vi "test1-LocalExternalStatusRegistration.vi"(8 "error in (no error)":errorcluster, 11 "TestCase in":refnum<class "testcase-CSMBroadcast.lvclass">) -> (0 "error out":errorcluster, 3 "TestCase out":refnum<class "testcase-CSMBroadcast.lvclass">)   [LabVIEW 2017, in "testcase-CSMBroadcast.lvclass"]
uses:
  testcase-CSMBroadcast.lvclass
  0b17d103-e67b-41be-a9eb-a2ee1311ff1f.vi
  5999693e-4f8a-4b34-ae87-f34dff5771be.vi
  52a2a10a-a04b-4bad-8df4-e1eb944f47cc.vi
  826f03dd-b4b5-4c6b-9085-8edf6da4f43b.vi
  src/user.lib/_NEVSTOP/Communicable State Machine(CSM)/AdvanceAPI/CSM - Revert Arguments-Safe String.vi
  src/user.lib/_NEVSTOP/Communicable State Machine(CSM)/AdvanceAPI/CSM - Make String Arguments Safe.vi
  src/user.lib/_NEVSTOP/Communicable State Machine(CSM)/AdvanceAPI/CSM - Break Down Multiple States String.vi
  src/user.lib/_NEVSTOP/Communicable State Machine(CSM)/AdvanceAPI/CSM - Keywords.vi
  src/user.lib/_NEVSTOP/Communicable State Machine(CSM)/_Polymophic/CSM - Replace Marks in Messages.vi
  src/user.lib/_NEVSTOP/Communicable State Machine(CSM)/AdvanceAPI/CSM - Get Module Attribute.vi
  src/user.lib/_NEVSTOP/Communicable State Machine(CSM)/_Shared/Trim Single-line Text.vi
  <vilib>/addons/_JKI Toolkits/VI Tester/TestCase.llb/TestCase.lvclass
  src/user.lib/_NEVSTOP/Communicable State Machine(CSM)/Communicable State Machine.lvlib
  C:/Program Files (x86)/National Instruments/LabVIEW 2017/vi.lib/addons/_JKI Toolkits/VI Tester/TestCase.llb/TestCase.lvclass
panel:
  out "One-Shot Unregistrations":string
  out "Waited (ms)":u32
  out "One-Shot Registrations":string
  out "LoopCount 2":i32
  out "State History":string
  out "LoopCount":i32
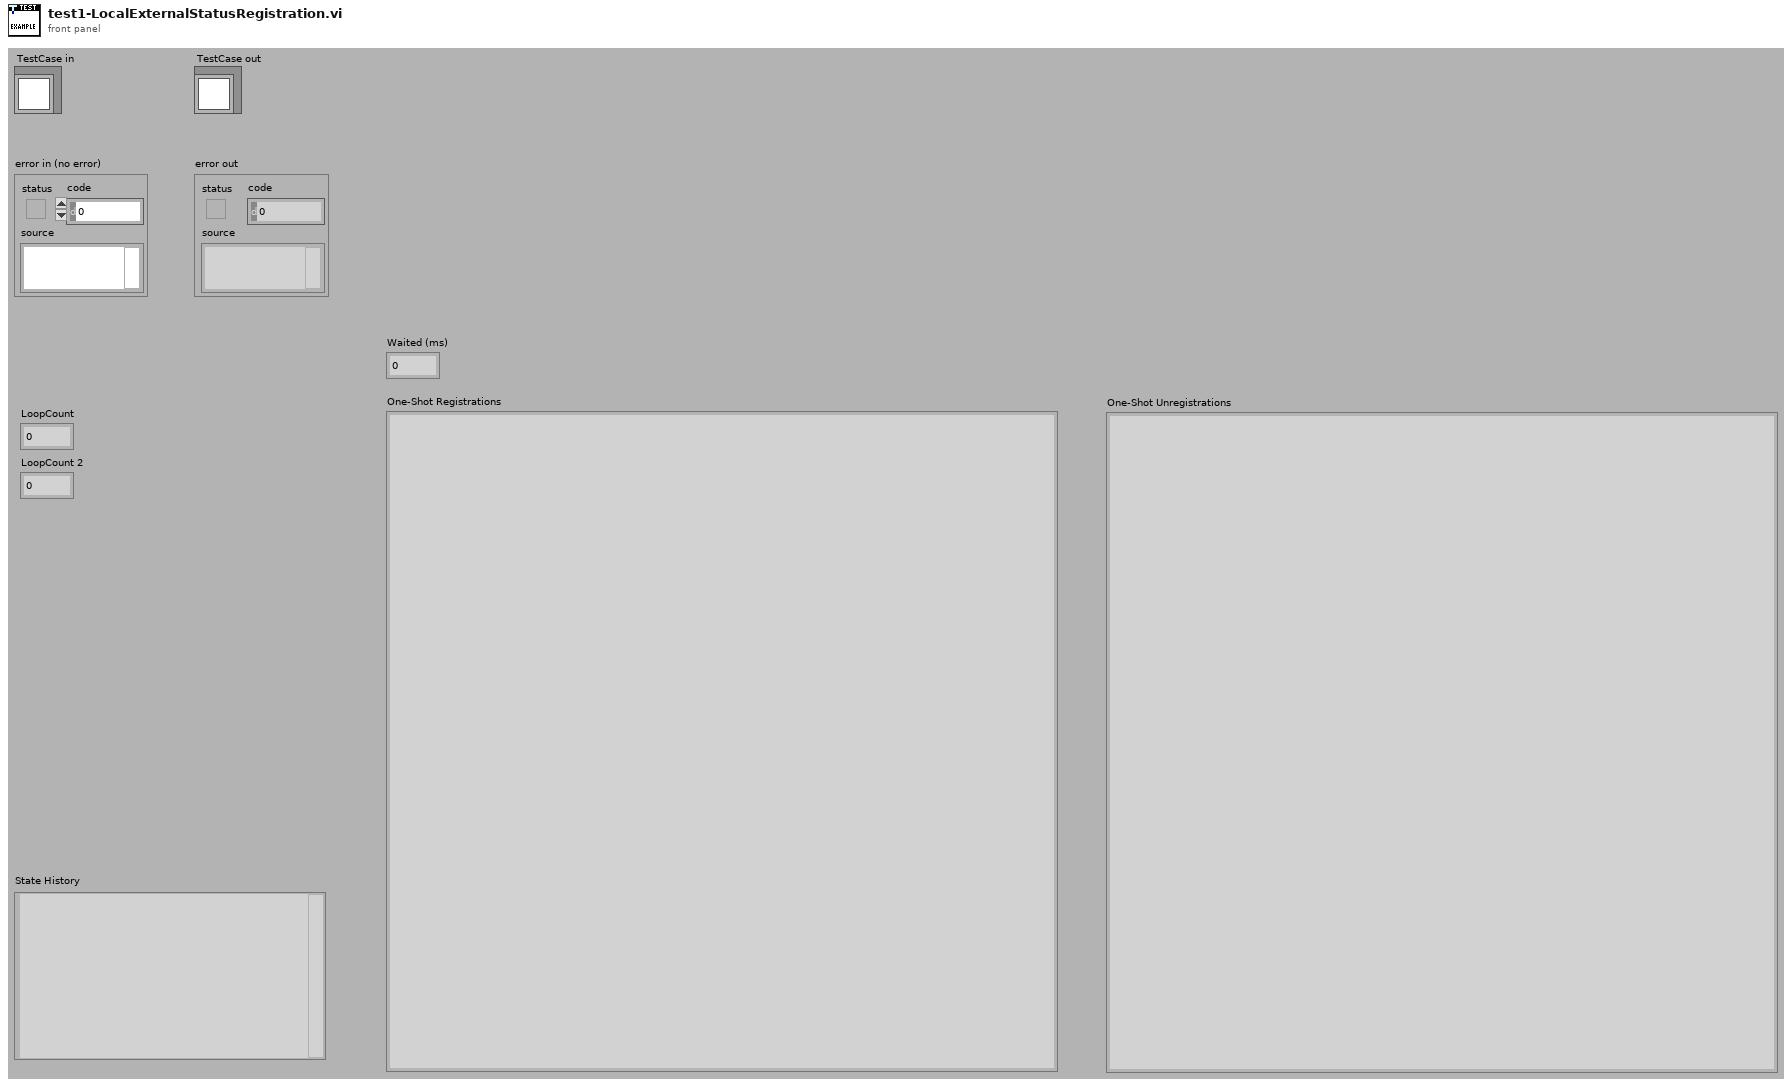
[diagram p1: front panel]
types:
  T1 = enum32{"Invalid", "Standard", "Closed", "Hidden", "Minimized", "Maximized"}
  T2 = enum32{"invalid app kind", "Development System", "Run Time System", "Student Edition", "Embedded LabVIEW", "Evaluation", "Custom"}
  T3 = typedef "Communicable State Machine.lvlib/_CSM_Response Source Message.ctl" = cluster{"‘State":string, "’Arguments":string, "’Error":errorcluster}
  T4 = cluster{"Current VI Reference":refnum<vi>, "Close Panel on Exit?":bool}
  T5 = cluster{"Core":cluster{"Current VI Reference":refnum<vi>, "Close Panel on Exit?":bool}, "Your Boolean data":bool, "Your string data":string}
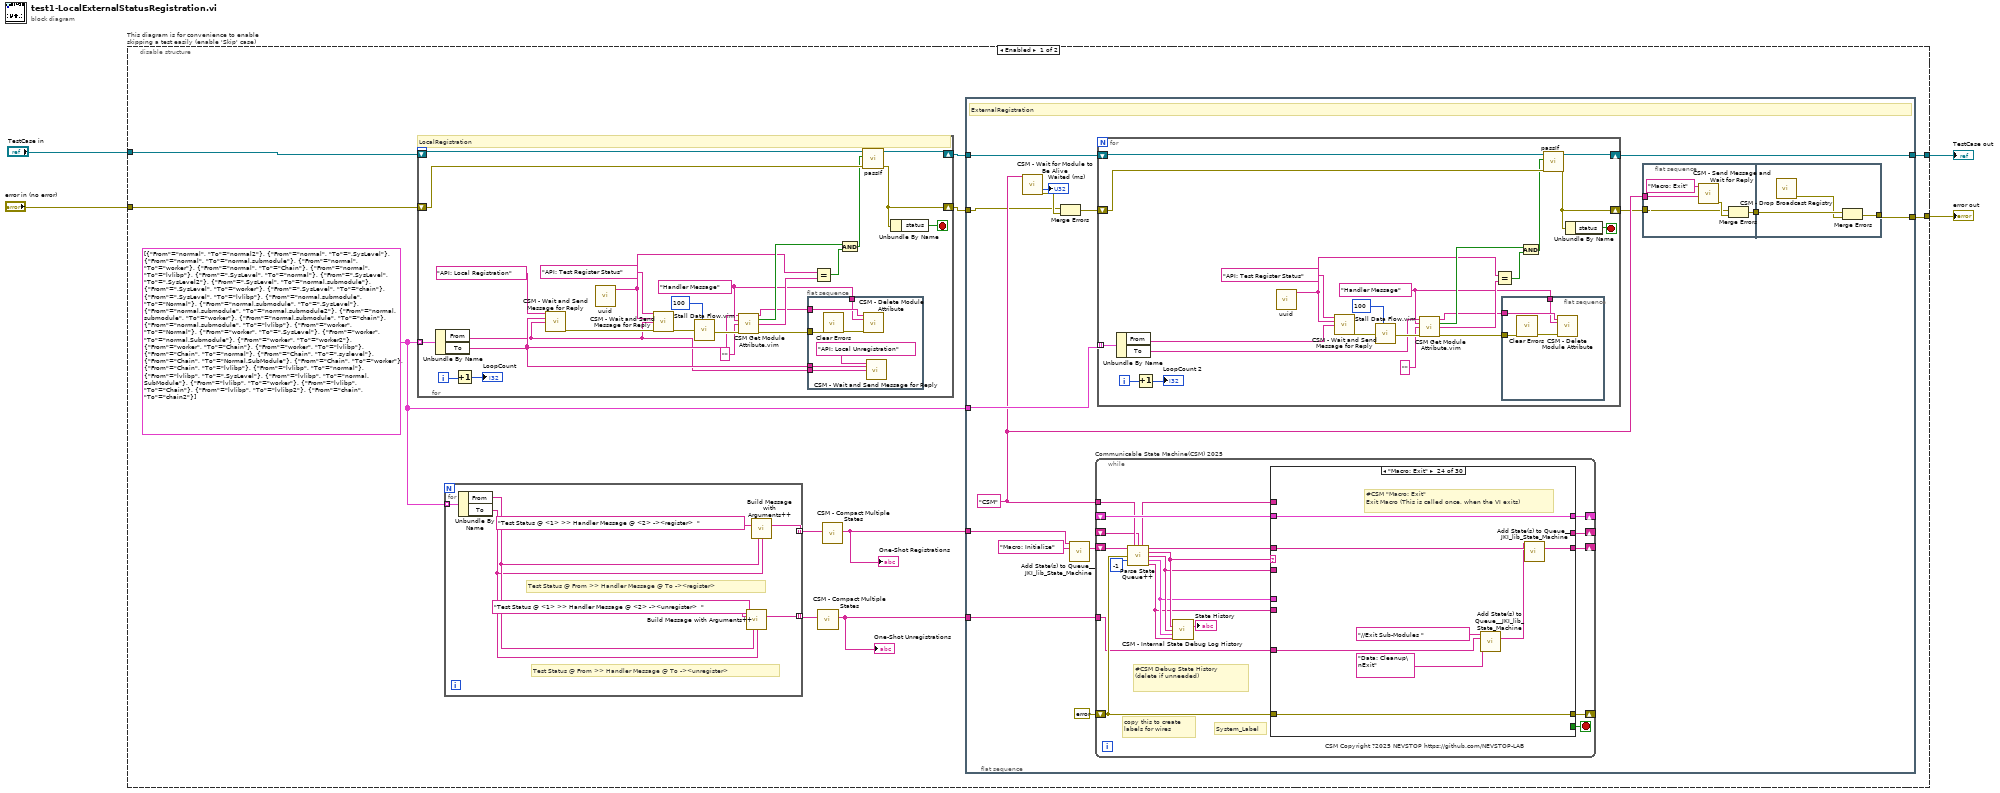
[diagram p0: block diagram]
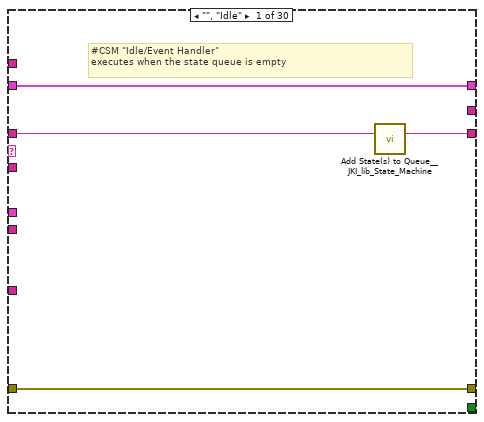
[diagram p2: hidden frame]
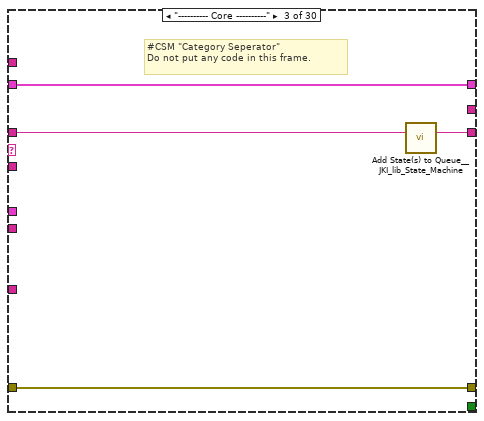
[diagram p4: hidden frame]
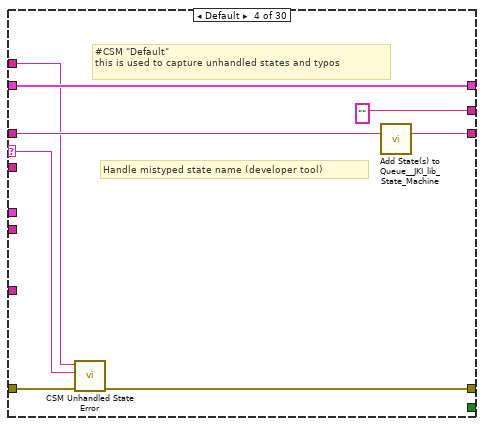
[diagram p5: hidden frame]
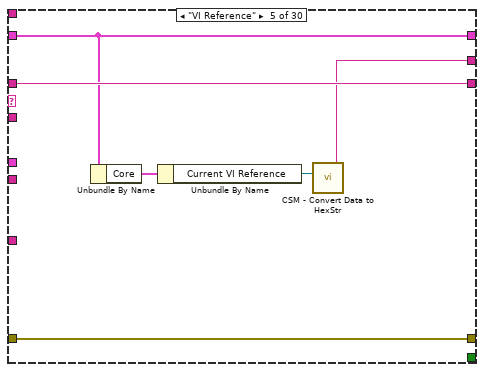
[diagram p6: hidden frame]
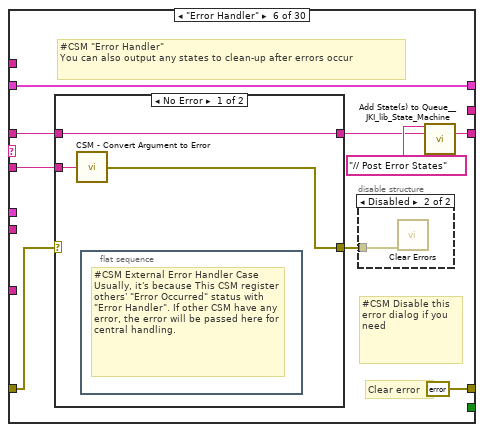
[diagram p7: hidden frame]
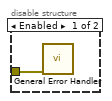
[diagram p8: hidden frame]
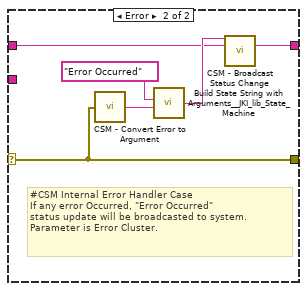
[diagram p9: hidden frame]
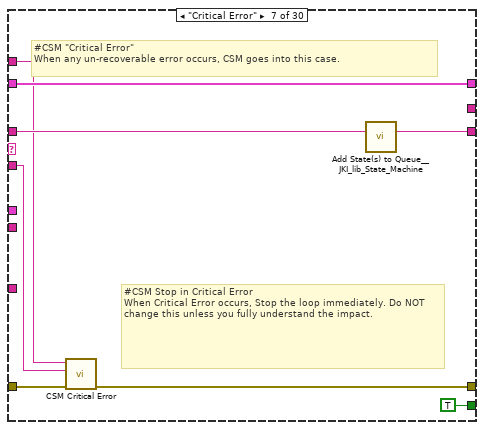
[diagram p10: hidden frame]
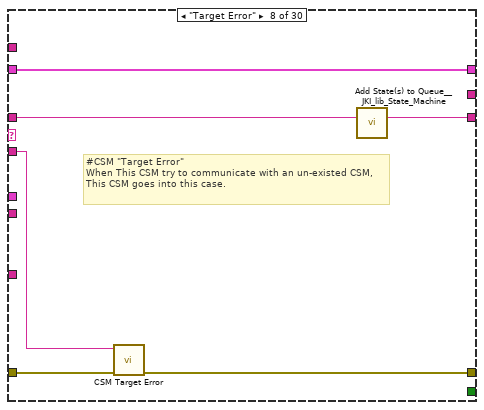
[diagram p11: hidden frame]
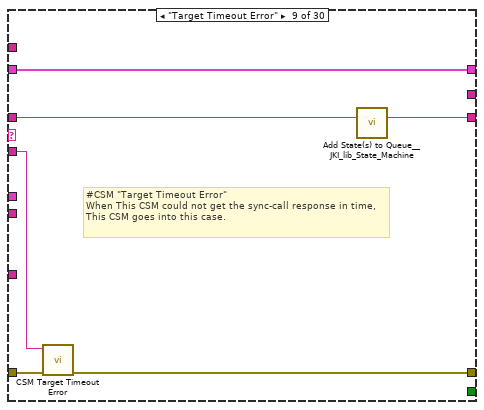
[diagram p12: hidden frame]
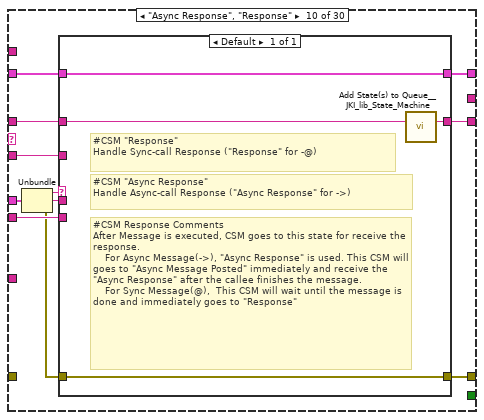
[diagram p13: hidden frame]
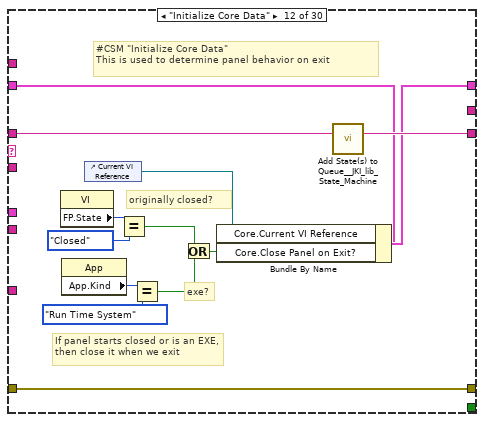
[diagram p15: hidden frame]
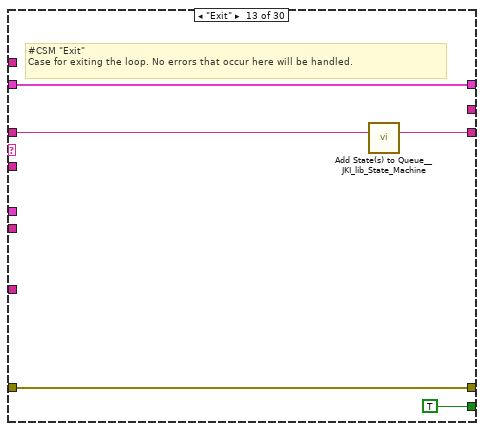
[diagram p16: hidden frame]
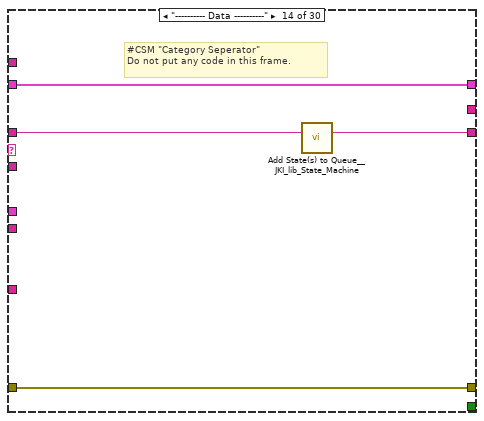
[diagram p17: hidden frame]
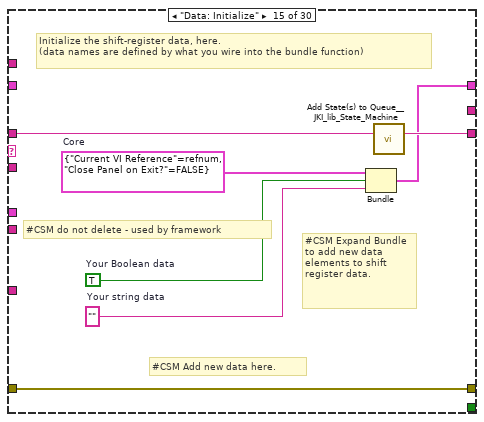
[diagram p18: hidden frame]
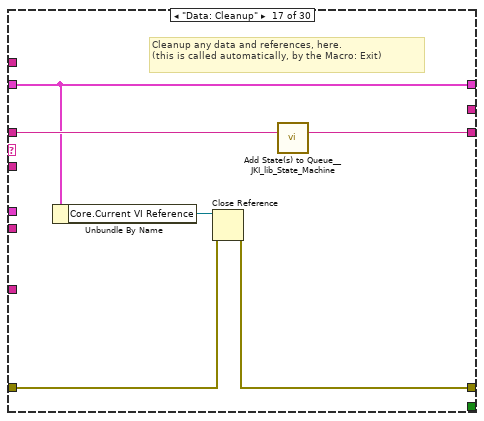
[diagram p20: hidden frame]
diagram:
  n1 = disable-structure "This diagram is for convenience to enable skipping a test easily (enable 'Skip' case)" shown="Enabled" {
    disable-tunnel: "TestCase in" -> [w14 w386]
    disable-tunnel: [w12 w384] -> w1
    disable-tunnel: [w5 w385] -> w3
    disable-tunnel: "error in (no error)" -> [w15 w383]
    frame Enabled {
      w10 = cluster{"From":string, "To":string}[] [{"From"="normal", "To"="normal2"}, {"From"="normal", "To"=".SysLevel"}, {"From"="normal", "To"="normal.submodule"}, {"From"="normal", "To"="worker"}, {"From"="normal", "To"="Chain"}, {"From"="normal", "To"="lvlibp"}, {"From"=".SysLevel", "To"="normal"}, {"From"=".SysLevel", "To"=".SysLevel2"}, {"From"=".SysLevel", "To"="normal.submodule"}, {"From"=".SysLevel", "To"="worker"}, {"From"=".SysLevel", "To"="chain"}, {"From"=".SysLevel", "To"="lvlibp"}, {"From"="normal.submodule", "To"="Normal"}, {"From"="normal.submodule", "To"=".SysLevel"}, {"From"="normal.submodule", "To"="normal.submodule2"}, {"From"="normal.submodule", "To"="worker"}, {"From"="normal.submodule", "To"="chain"}, {"From"="normal.submodule", "To"="lvlibp"}, {"From"="worker", "To"="Normal"}, {"From"="worker", "To"=".SysLevel"}, {"From"="worker", "To"="normal.Submodule"}, {"From"="worker", "To"="worker2"}, {"From"="worker", "To"="Chain"}, {"From"="worker", "To"="lvlibp"}, {"From"="Chain", "To"="normal"}, {"From"="Chain", "To"=".syslevel"}, {"From"="Chain", "To"="Normal.SubModule"}, {"From"="Chain", "To"="worker"}, {"From"="Chain", "To"="lvlibp"}, {"From"="lvlibp", "To"="normal"}, {"From"="lvlibp", "To"=".SysLevel"}, {"From"="lvlibp", "To"="normal.SubModule"}, {"From"="lvlibp", "To"="worker"}, {"From"="lvlibp", "To"="Chain"}, {"From"="lvlibp", "To"="lvlibp2"}, {"From"="chain", "To"="chain2"}]
      n2 = for {
        shift-right: [w24] -> w11
        shift-left: w15 -> [w25]
        shift-right: [w26] -> w13
        shift-left: w14 -> [w27]
        tunnel: w10 -> [w38] mode=indexing
        i -> [w40]
        stop <- w23 stop-if-true
        w18 = "Handler Message" ("To")
        # "LocalRegistration"
        n3 = Unbundle By Name(w38) -> ("From"=w16:string, "To"=w17:string)
        n4 = Increment(x=w40) -> (x+1=→"LoopCount":i32)
        n5 = call "CSM - Wait and Send Message for Reply.vi"("State"="API: Local Registration", "Arguments (\"\")"=w17, "Target Module"=w16) -> ("error out"=w35:errorcluster)  [unwired: 9 in, 3 out]
        n6 = call "uuid.vi"() -> ("UUID"=w29:string)  [unwired: 11 in]
        n7 = call "CSM - Wait and Send Message for Reply.vi"("State"="API: Test Register Status", "Arguments (\"\")"=w29, "Target Module"=w16, "Error In (No Error)"=w35) -> ("error out"=w34:errorcluster)  [unwired: 8 in, 3 out]
        n8 = call "Stall Data Flow.vim"("value in"=w34, "milliseconds to wait"=u32 100) -> ("value out"=w32:errorcluster)  [unwired: 1 out]
        n9 = call "CSM Get Module Attribute.vim"("CSM Name"=w17, "Attribute"=w18, "Default Value (Empty Variant)"="", "Error In"=w32) -> ("CSM Name (Dup)"=w19:string, "Found"=w31:bool, "Value"=w28:string, "error out"=w20:errorcluster)  [unwired: 7 in, 1 out]
        n10 = flat-sequence {
          tunnel: w20 -> [w46]
          tunnel: w19 -> [w45]
          tunnel: w18 -> [w44]
          tunnel: w17 -> [w42]
          tunnel: w16 -> [w41]
          frame #0 {
            n11 = call <vilib>:"Clear Errors.vi"("error in (no error)"=w46) -> ("error out"=w47:errorcluster)  [unwired: 5 in, 1 out]
            n12 = call "CSM - Delete Module Attribute.vi"("CSM Name"=w45, "Attribute"=w44, "Error In"=w47) -> ()  [unwired: 9 in, 4 out]
            n13 = call "CSM - Wait and Send Message for Reply.vi"("State"="API: Local Unregistration", "Arguments (\"\")"=w42, "Target Module"=w41) -> ()  [unwired: 9 in, 4 out]
          }
        }
        n14 = Equal?(x=w29, y=w28) -> (x = y?=w22:bool)
        n15 = And(x=w31, y=w22) -> (x .and. y?=w21:bool)
        n16 = call-dynamic "passIf.vi"("error in (no error)"=w25, "pass"=w21, "TestCase in"=w27) -> ("error out"=w24:errorcluster, "TestCase out"=w26:refnum<class "testcase-CSMBroadcast.lvclass">)  [unwired: 7 in]
        n17 = Unbundle By Name(w24) -> ("status"=w23:bool)
      }
      n18 = for {
        tunnel: w10 -> [w53] mode=indexing
        tunnel: [w52] -> w9 mode=indexing
        tunnel: [w48] -> w7 mode=indexing
        # "Test Status @ From >> Handler Message @ To -><unregister>"
        # "Test Status @ From >> Handler Message @ To -><register>"
        n19 = Unbundle By Name(w53) -> ("From"=w50:string, "To"=w49:string)
        n20 = call-poly "Build Message with Arguments++.vi"("States With Replace Token"="Test Status @ <1> >> Handler Message @ <2> -><unregister>  " ("State"), "<1>"=w50, "<2>"=w49) -> ("States"=w48:string)  [unwired: 12 in]
        n21 = call-poly "Build Message with Arguments++.vi"("States With Replace Token"="Test Status @ <1> >> Handler Message @ <2> -><register>  " ("State"), "<1>"=w50, "<2>"=w49) -> ("States"=w52:string)  [unwired: 12 in]
      }
      n22 = call "CSM - Compact Multiple States.vi"("Multiple States"=w7) -> ("States"=w6:string)  [unwired: 9 in]
      "One-Shot Unregistrations" <- w6
      n23 = call "CSM - Compact Multiple States.vi"("Multiple States"=w9) -> ("States"=w8:string)  [unwired: 9 in]
      "One-Shot Registrations" <- w8
      n24 = flat-sequence {
        tunnel: w13 -> [w67]
        tunnel: [w66] -> w12
        tunnel: w11 -> [w59]
        tunnel: w10 -> [w65]
        tunnel: w8 -> [w63]
        tunnel: w6 -> [w57]
        tunnel: [w55] -> w5
        frame #0 {
          w62 = "CSM" ("Name (\"\" to Use UUID)")
          # "ExternalRegistration"
          n25 = call "CSM - Wait for Module to Be Alive.vi"("CSM Name"=w62) -> ("Waited (ms)"=→"Waited (ms)":u32, "error out"=w64:errorcluster)  [unwired: 12 in, 1 out]
          n26 = Merge Errors(w59, w64) -> (w60:errorcluster)
          n27 = call <vilib>:"Add State(s) to Queue__JKI_lib_State_Machine.vi"("State(s) in Front (\"\")"=w63, "State(s) in (\"\")"="Macro: Initialize" ("Init State(\"Macro: Initialize\")")) -> ("States Out"=w68:string)  [unwired: 13 in]
          n28 = while "Communicable State Machine(CSM) 2025" {
            shift-right: [w119] -> _
            shift-left: _ -> [w118]
            shift-right: [w122] -> _
            shift-left: errorcluster {"status"=FALSE, "code"=0, "source"=""} ("error out") -> [w117]
            shift-right: [w121] -> _
            shift-left: w68 -> [w123]
            tunnel: w62 -> [w115]
            shift-right: [w116] -> _
            shift-left: _ -> [w109]
            tunnel: w57 -> [w106]
            stop <- w120 stop-if-true
            # "#CSM Debug State History\n(delete if unneeded)"
            # "copy this to create labels for wires"
            # "System_Label"
            # "CSM Copyright ?2025 NEVSTOP https://github.com/NEVSTOP-LAB"
            n29 = call "Parse State Queue++.vi"("State Queue"=w123, "Name (\"\" to Use UUID)"=w115, "Response Arguments"=w109, "Previous Error"=w117, "Dequeue (1 ms)"=-1 ("Timeout")) -> ("Name Used"=w110:string, "Remaining States"=w124:string, "Current State"=w114:string, "Arguments"=w113:string, "Additional Information"=w112:T3, "Source CSM"=w111:string)  [unwired: 5 in]
            n30 = call "CSM - Internal State Debug Log History.vi"("State"=w114, "Arguments (\"\")"=w113, ">> Response Source Message >>"=w112, "Source (\"\")"=w111) -> ("Debug Log"=→"State History":string)  [unwired: 11 in]
            n31 = case shown="\"Macro: Exit\"" w114 {
              selector: w114 -> [_ _ _ w138 _ _ _ _ _ _ _ _ _ _ _ _ _ _ _ _ _ _ _ _ _ _ _ _ _ _]
              tunnel: w124 -> [w125 w130 w135 w142 w148 w154 w175 w181 w187 w195 w206 w220 w225 w229 w236 w238 w245 w249 w253 w259 w274 w343 w348 w356 w358 w362 w367 w374 w378 w382]
              tunnel: w113 -> [_ _ _ _ _ w153 w171 w180 w185 w194 _ _ _ _ _ _ _ _ _ w254 w268 _ _ _ _ _ w365 _ _ _]
              tunnel: w118 -> [w126 w129 w132 w140 w147 w157 w176 w182 w188 w197 w205 w213 w223 w226 _ w237 w240 w246 w251 w257 w270 w340 w345 w353 w357 w361 w366 w371 w375 w379]
              tunnel: [w127 w131 w133 w136 w149 errorcluster {"status"=FALSE, "code"=0, "source"=""} ("error out") w172 w178 w184 w200 w207 w217 w222 w227 w233 w239 w241 w247 w250 w255 w271 w341 w346 w354 w359 w363 w368 w372 w376 w380] -> w122
              tunnel: w117 -> [w127 w131 w133 w143 w149 w155 w177 w179 w186 _ w207 w217 w222 w227 w233 w239 w242 w247 w250 w256 w272 w341 w346 w354 w359 w363 w368 w372 w376 w380]
              tunnel: [w128 w130 w134 w141 w148 w150 w174 w183 w189 w196 w206 w219 w224 w228 w235 w238 w244 w248 w252 w258 w273 w342 w347 w355 w358 w362 w367 w373 w377 w381] -> w121
              tunnel: [_ _ _ _ _ _ TRUE _ _ _ _ _ TRUE _ _ _ _ _ _ _ _ _ _ _ _ _ _ _ _ _] -> w120
              tunnel: [w126 w129 w132 w140 w147 w157 w176 w182 w188 w198 w205 w218 w223 w226 w234 w237 w240 w246 w251 w257 w270 w340 w345 w353 w357 w361 w366 w371 w375 w379] -> w119
              tunnel: w111 -> [_ _ _ _ _ _ _ _ _ w192 _ _ _ _ _ _ _ _ _ _ _ _ _ _ _ _ _ _ _ _]
              tunnel: w112 -> [_ _ _ _ _ _ _ _ _ w199 _ _ _ _ _ _ _ _ _ _ _ _ _ _ _ _ _ _ _ _]
              tunnel: [_ _ _ "" w144 _ _ _ _ _ _ _ _ _ _ _ _ _ _ _ _ _ _ _ _ "API1 Response" w364 _ _ _] -> w116
              tunnel: w110 -> [_ _ _ w137 _ _ w170 _ _ _ _ _ _ _ _ _ _ _ _ _ _ _ _ _ _ _ _ _ _ _]
              tunnel: w106 -> [_ _ _ _ _ _ _ _ _ _ _ _ _ _ _ _ _ _ _ _ _ _ _ w349 _ _ _ _ _ _]
              frame "", "Idle" {
                # "#CSM \"Idle/Event Handler\"\nexecutes when the state queue is empty"
                n32 = call <vilib>:"Add State(s) to Queue__JKI_lib_State_Machine.vi"("State(s) in (\"\")"=w125) -> ("States Out"=w128:string)  [unwired: 14 in]
              }
              frame "CSM Documentation" {
                # "#CSM README FIRST\n\nCommunicable State Machine(CSM) is a LabVIEW application framework that builds upon JKI State Machine(JKISM). It follows the pattern of JKISM and extends the keywords to describe message communication between modules, including concepts such as Sync-Message, Async-Message, Subscription/Unsubscription of status - essential elements for creating reusable code modules. For more information, please visit the CSM wiki: https://nevstop-lab.github.io/CSM-Wiki/\n\nFor instructions on JKI State Machine, visit: http://jki.net/state-machine/\nFor information about CSM, visit: https://github.com/NEVSTOP-LAB"
                # "#CSM \"Documentation\"\nCase for holding CSM Documenation"
              }
              frame "---------- Core ----------" {
                # "#CSM \"Category Seperator\"\nDo not put any code in this frame."
                n33 = call <vilib>:"Add State(s) to Queue__JKI_lib_State_Machine.vi"("State(s) in (\"\")"=w135) -> ("States Out"=w134:string)  [unwired: 14 in]
              }
              frame Default {
                # "#CSM \"Default\"\nthis is used to capture unhandled states and typos"
                # "Handle mistyped state name (developer tool)"
                n34 = call "CSM Unhandled State Error.vi"("error in (no error)"=w143, "Undefined State"=w138, "CSM Name"=w137) -> ("error out"=w136:errorcluster)  [unwired: 8 in]
                n35 = call <vilib>:"Add State(s) to Queue__JKI_lib_State_Machine.vi"("State(s) in (\"\")"=w142) -> ("States Out"=w141:string)  [unwired: 14 in]
              }
              frame "VI Reference" {
                n36 = Unbundle By Name(w147) -> ("Core"=w146:T4)
                n37 = Unbundle By Name(w146) -> ("Current VI Reference"=w145:refnum<vi>)
                n38 = call "CSM - Convert Data to HexStr.vi"("Variant"=w145) -> ("HEX String (0-9,A-F)"=w144:string)  [unwired: 8 in]
              }
              frame "Error Handler" {
                # "#CSM Disable this error dialog if you need"
                # "#CSM \"Error Handler\"\nYou can also output any states to clean-up after errors occur"
                # "Clear error"
                n39 = case shown="No Error" w155 {
                  selector: w155 -> [_ w164]
                  tunnel: [w163 w166] -> w151
                  tunnel: w154 -> [w163 w165]
                  tunnel: w153 -> [w162 _]
                  tunnel: [w161 w164] -> w156
                  frame No Error {
                    n40 = call "CSM - Convert Argument to Error.vi"("Argument"=w162) -> ("Error"=w161:errorcluster)  [unwired: 4 in]
                    n41 = flat-sequence {
                      frame #0 {
                        # "#CSM External Error Handler Case\nUsually, it's because This CSM register others' \"Error Occurred\" status with \"Error Handler\". If other CSM have any error, the error will be passed here for central handling."
                      }
                    }
                  }
                  frame Error {
                    # "#CSM Internal Error Handler Case \nIf any error Occurred, \"Error Occurred\" \nstatus update will be broadcasted to system.\nParameter is Error Cluster."
                    n42 = call "CSM - Convert Error to Argument.vi"("Error"=w164) -> ("Argument"=w168:string)  [unwired: 4 in]
                    n43 = call <vilib>:"Build State String with Arguments__JKI_lib_State_Machine.vi"("Arguments (\"\")"=w168, "State"="Error Occurred" ("Status with Arguments")) -> ("State with Arguments"=w167:string)  [unwired: 4 in]
                    n44 = call "CSM - Broadcast Status Change.vi"("Status With Arguments"=w167, "State Queue"=w165) -> ("Remaining States"=w166:string)  [unwired: 13 in]
                  }
                }
                n45 = disable-structure shown="Disabled" {
                  disable-tunnel: w156 -> [w159 w160]
                  frame Enabled {
                    n46 = call <vilib>:"General Error Handler.vi"("error in (no error)"=w159) -> ()  [unwired: 10 in, 5 out]
                  }
                  frame Disabled {
                    n47 = call <vilib>:"Clear Errors.vi"("error in (no error)"=w160) -> ()  [unwired: 5 in, 2 out]
                  }
                }
                n48 = call <vilib>:"Add State(s) to Queue__JKI_lib_State_Machine.vi"("State(s) in Front (\"\")"="// Post Error States", "State(s) in (\"\")"=w151) -> ("States Out"=w150:string)  [unwired: 13 in]
              }
              frame "Critical Error" {
                # "#CSM Stop in Critical Error\nWhen Critical Error occurs, Stop the loop immediately. Do NOT change this unless you fully understand the impact."
                # "#CSM \"Critical Error\"\nWhen any un-recoverable error occurs, CSM goes into this case."
                n49 = call "CSM Critical Error.vi"("error in (no error)"=w177, "Arugments (As Reason)"=w171, "CSM Name"=w170) -> ("error out"=w172:errorcluster)  [unwired: 8 in]
                n50 = call <vilib>:"Add State(s) to Queue__JKI_lib_State_Machine.vi"("State(s) in (\"\")"=w175) -> ("States Out"=w174:string)  [unwired: 14 in]
              }
              frame "Target Error" {
                # "#CSM \"Target Error\"\nWhen This CSM try to communicate with an un-existed CSM, This CSM goes into this case."
                n51 = call "CSM Target Error.vi"("error in (no error)"=w179, "Arguments (As CSM Name)"=w180) -> ("error out"=w178:errorcluster)  [unwired: 9 in]
                n52 = call <vilib>:"Add State(s) to Queue__JKI_lib_State_Machine.vi"("State(s) in (\"\")"=w181) -> ("States Out"=w183:string)  [unwired: 14 in]
              }
              frame "Target Timeout Error" {
                # "#CSM \"Target Timeout Error\"\nWhen This CSM could not get the sync-call response in time, This CSM goes into this case."
                n53 = call "CSM Target Timeout Error.vi"("error in (no error)"=w186, "Arguments (As CSM Name)"=w185) -> ("error out"=w184:errorcluster)  [unwired: 9 in]
                n54 = call <vilib>:"Add State(s) to Queue__JKI_lib_State_Machine.vi"("State(s) in (\"\")"=w187) -> ("States Out"=w189:string)  [unwired: 14 in]
              }
              frame "Async Response", "Response" {
                n55 = Unbundle(w199) -> ("‘State"=w193:string, "’Arguments"=w191:string, "’Error"=w190:errorcluster)
                n56 = case shown="Default" w193 {
                  tunnel: [w204] -> w200
                  tunnel: w190 -> [w204]
                  tunnel: [w203] -> w198
                  tunnel: w197 -> [w203]
                  tunnel: [w201] -> w196
                  tunnel: w195 -> [w202]
                  tunnel: w194 -> [_]
                  tunnel: w192 -> [_]
                  tunnel: w191 -> [_]
                  frame Default {
                    # "#CSM Response Comments\nAfter Message is executed, CSM goes to this state for receive the response.\n    For Async Message(->), \"Async Response\" is used. This CSM will goes to \"Async Message Posted\" immediately and receive the \"Async Response\" after the callee finishes the message.\n    For Sync Message(@),  This CSM will wait until the message is done and immediately goes to \"Response\""
                    # "#CSM \"Async Response\"\nHandle Async-call Response (\"Async Response\" for ->)"
                    # "#CSM \"Response\"\nHandle Sync-call Response (\"Response\" for -@)"
                    n57 = call <vilib>:"Add State(s) to Queue__JKI_lib_State_Machine.vi"("State(s) in (\"\")"=w202) -> ("States Out"=w201:string)  [unwired: 14 in]
                  }
                }
              }
              frame "Async Message Posted" {
                # "#CSM \"Async Message Posted\"\nAfter Async Message is posted (-> or ->| ), CSM goes to this state for post-action.\nYou can use Argument - State to tell which Async Message is called."
              }
              frame "Initialize Core Data" {
                # "#CSM \"Initialize Core Data\"\nThis is used to determine panel behavior on exit"
                # "originally closed?"
                # "exe?"
                # "If panel starts closed or is an EXE, then close it when we exit"
                n58 = property class="VI"() -> ("FP.State"=w210:T1)  [unwired: 2 in, 2 out]
                n59 = property class="App"() -> ("App.Kind"=w216:T2)  [unwired: 2 in, 2 out]
                n60 = control-ref of="Current VI Reference"() -> (w211:refnum<vi>)
                n61 = Equal?(x=w210, y=T1."Closed" ("Front Panel Window:State")) -> (x = y?=w208:bool)
                n62 = Equal?(x=w216, y=T2."Run Time System" ("Application:Kind")) -> (x = y?=w214:bool)
                n63 = Or(x=w208, y=w214) -> (x .or. y?=w212:bool)
                n64 = Bundle By Name(cluster=w213, "Core.Current VI Reference"=w211, "Core.Close Panel on Exit?"=w212) -> (w218:T5)
                n65 = call <vilib>:"Add State(s) to Queue__JKI_lib_State_Machine.vi"("State(s) in (\"\")"=w220) -> ("States Out"=w219:string)  [unwired: 14 in]
              }
              frame "Exit" {
                # "#CSM \"Exit\"\nCase for exiting the loop. No errors that occur here will be handled."
                n66 = call <vilib>:"Add State(s) to Queue__JKI_lib_State_Machine.vi"("State(s) in (\"\")"=w225) -> ("States Out"=w224:string)  [unwired: 14 in]
              }
              frame "---------- Data ----------" {
                # "#CSM \"Category Seperator\"\nDo not put any code in this frame."
                n67 = call <vilib>:"Add State(s) to Queue__JKI_lib_State_Machine.vi"("State(s) in (\"\")"=w229) -> ("States Out"=w228:string)  [unwired: 14 in]
              }
              frame "Data: Initialize" {
                w230 = T4 {"Current VI Reference"=refnum, "Close Panel on Exit?"=FALSE}  # Core
                w232 = TRUE  # Your Boolean data
                w231 = ""  # Your string data
                # "#CSM do not delete - used by framework"
                # "#CSM Expand Bundle to add new data elements to shift register data."
                # "#CSM Add new data here."
                # "Initialize the shift-register data, here.\n(data names are defined by what you wire into the bundle function)"
                n68 = Bundle("Core"=w230, "Your Boolean data"=w232, "Your string data"=w231) -> (w234:T5)  [unwired: 1 in]
                n69 = call <vilib>:"Add State(s) to Queue__JKI_lib_State_Machine.vi"("State(s) in (\"\")"=w236) -> ("States Out"=w235:string)  [unwired: 14 in]
              }
              frame "Data: Update Indicators" {
              }
              frame "Data: Cleanup" {
                # "Cleanup any data and references, here.\n(this is called automatically, by the Macro: Exit)"
                n70 = Unbundle By Name(w240) -> ("Core.Current VI Reference"=w243:refnum<vi>)
                n71 = Close Reference(reference=w243, error in (no error)=w242) -> (error out=w241:errorcluster)
                n72 = call <vilib>:"Add State(s) to Queue__JKI_lib_State_Machine.vi"("State(s) in (\"\")"=w245) -> ("States Out"=w244:string)  [unwired: 14 in]
              }
              frame "---------- UI ----------" {
                # "#CSM \"Category Seperator\"\nDo not put any code in this frame."
                n73 = call <vilib>:"Add State(s) to Queue__JKI_lib_State_Machine.vi"("State(s) in (\"\")"=w249) -> ("States Out"=w248:string)  [unwired: 14 in]
              }
              frame "UI: Initialize" {
                # "#CSM \"UI: Initialize\"\nInitialize the User Interface, here.\n(this is called automatically, by the Macro: Init)"
                n74 = call <vilib>:"Add State(s) to Queue__JKI_lib_State_Machine.vi"("State(s) in (\"\")"=w253) -> ("States Out"=w252:string)  [unwired: 14 in]
              }
              frame "UI: Cursor Set" {
                # "#CSM \"UI: Cursor Set\"\nSet and Unset Cursor Busy.\n(Usage: \"UI: Cursor Set >> Busy|Idle\")"
                # "Argument"
                n75 = disable-structure shown="TARGET_TYPE!=Windows" {
                  disable-tunnel: w256 -> [w262 w267]
                  disable-tunnel: [w261 w267] -> w255
                  disable-tunnel: w254 -> [w260 _]
                  frame condition #0 (active) {
                    n76 = case shown="\"Idle\", Default" w260 {
                      tunnel: w262 -> [w264 w266]
                      tunnel: [w263 w265] -> w261
                      frame "Idle", Default {
                        n77 = call <vilib>:"Unset Busy.vi"("error in (no error)"=w264) -> ("error out"=w263:errorcluster)  [unwired: 10 in]
                      }
                      frame "Busy" {
                        n78 = call <vilib>:"Set Busy.vi"("error in (no error)"=w266) -> ("error out"=w265:errorcluster)  [unwired: 9 in, 1 out]
                      }
                    }
                  }
                  frame condition #1 {
                  }
                }
                n79 = call <vilib>:"Add State(s) to Queue__JKI_lib_State_Machine.vi"("State(s) in (\"\")"=w259) -> ("States Out"=w258:string)  [unwired: 14 in]
              }
              frame "UI: Front Panel State" {
                # "#CSM \"UI: Front Panel State\"\nSet Front Panel Open or Closed\n(Usage: \"UI: Front Panel State >> Open|Close\")"
                # "Argument"
                n80 = Unbundle By Name(w270) -> ("Core.Current VI Reference"=w269:refnum<vi>)
                n81 = call <vilib>:"Add State(s) to Queue__JKI_lib_State_Machine.vi"("State(s) in (\"\")"=w274) -> ("States Out"=w273:string)  [unwired: 14 in]
                n82 = case shown="\"Close\", \"Closed\"" w268 {
                  tunnel: w272 -> [w280 w295 w306 w319 w332]
                  tunnel: [w282 w296 w308 w321 w334] -> w271
                  tunnel: w269 -> [w281 w293 w307 w320 w333]
                  frame "Open", "Standard", Default {
                    w275 = T1."Standard" ("State")
                    n83 = property class="VI"(reference=w281, error in=w280) -> (reference out=w278:refnum<vi>, error out=w279:errorcluster, "FP.State"=w277:T1)
                    n84 = Not Equal?(x=w277, y=w275) -> (x != y?=w276:bool)
                    n85 = case shown="True" w276 {
                      tunnel: [w286 w288] -> w282
                      tunnel: w279 -> [w285 w288]
                      tunnel: w278 -> [w284 _]
                      tunnel: w275 -> [w283 _]
                      frame True {
                        n86 = invoke class="VI" method="FP.Open"(reference=w284, error in=w285, "Activate"=TRUE, "State"=w283) -> (error out=w286:errorcluster)  [unwired: 1 in, 4 out]
                      }
                      frame False {
                      }
                    }
                  }
                  frame "Close", "Closed" {
                    n87 = property class="VI"(reference=w293, error in=w295) -> (reference out=w292:refnum<vi>, error out=w294:errorcluster, "FP.State"=w290:T1)
                    n88 = Not Equal?(x=w290, y=T1."Closed" ("Front Panel Window:State")) -> (x != y?=w289:bool)
                    n89 = case shown="False" w289 {
                      tunnel: [w297 w300] -> w296
                      tunnel: w294 -> [w297 w299]
                      tunnel: w292 -> [_ w298]
                      frame False {
                      }
                      frame True {
                        n90 = invoke class="VI" method="FP.Close"(reference=w298, error in=w299) -> (error out=w300:errorcluster)  [unwired: 1 in, 2 out]
                      }
                    }
                  }
                  frame "Hidden", "Hide" {
                    w301 = T1."Hidden" ("State")
                    n91 = property class="VI"(reference=w307, error in=w306) -> (reference out=w304:refnum<vi>, error out=w305:errorcluster, "FP.State"=w303:T1)
                    n92 = Not Equal?(x=w303, y=w301) -> (x != y?=w302:bool)
                    n93 = case shown="True" w302 {
                      tunnel: [w312 w313] -> w308
                      tunnel: w305 -> [w311 w313]
                      tunnel: w304 -> [w310 _]
                      tunnel: w301 -> [w309 _]
                      frame True {
                        n94 = invoke class="VI" method="FP.Open"(reference=w310, error in=w311, "State"=w309) -> (error out=w312:errorcluster)  [unwired: 2 in, 4 out]
                      }
                      frame False {
                      }
                    }
                  }
                  frame "Minimize", "Minimized" {
                    w314 = T1."Minimized" ("State")
                    n95 = property class="VI"(reference=w320, error in=w319) -> (reference out=w317:refnum<vi>, error out=w318:errorcluster, "FP.State"=w316:T1)
                    n96 = Not Equal?(x=w316, y=w314) -> (x != y?=w315:bool)
                    n97 = case shown="True" w315 {
                      tunnel: [w325 w326] -> w321
                      tunnel: w318 -> [w324 w326]
                      tunnel: w317 -> [w323 _]
                      tunnel: w314 -> [w322 _]
                      frame True {
                        n98 = invoke class="VI" method="FP.Open"(reference=w323, error in=w324, "State"=w322) -> (error out=w325:errorcluster)  [unwired: 2 in, 4 out]
                      }
                      frame False {
                      }
                    }
                  }
                  frame "Maximize", "Maximized" {
                    w327 = T1."Maximized" ("State")
                    n99 = property class="VI"(reference=w333, error in=w332) -> (reference out=w330:refnum<vi>, error out=w331:errorcluster, "FP.State"=w329:T1)
                    n100 = Not Equal?(x=w329, y=w327) -> (x != y?=w328:bool)
                    n101 = case shown="True" w328 {
                      tunnel: [w338 w339] -> w334
                      tunnel: w331 -> [w337 w339]
                      tunnel: w330 -> [w336 _]
                      tunnel: w327 -> [w335 _]
                      frame True {
                        n102 = invoke class="VI" method="FP.Open"(reference=w336, error in=w337, "State"=w335) -> (error out=w338:errorcluster)  [unwired: 2 in, 4 out]
                      }
                      frame False {
                      }
                    }
                  }
                }
              }
              frame "---------- Macro ----------" {
                # "#CSM \"Category Seperator\"\nDo not put any code in this frame."
                n103 = call <vilib>:"Add State(s) to Queue__JKI_lib_State_Machine.vi"("State(s) in (\"\")"=w343) -> ("States Out"=w342:string)  [unwired: 14 in]
              }
              frame "Macro: Initialize" {
                # "#CSM \"Macro: Initialize\"\nInitialization Macro (This is called once, when the VI starts)"
                n104 = call <vilib>:"Add State(s) to Queue__JKI_lib_State_Machine.vi"("State(s) in Front (\"\")"="Data: Initialize\nInitialize Core Data\nData: Update Indicators", "State(s) in (\"\")"=w348) -> ("States Out"=w347:string)  [unwired: 13 in]
              }
              frame "Macro: Exit" {
                # "#CSM \"Macro: Exit\"\nExit Macro (This is called once, when the VI exits)"
                n105 = call <vilib>:"Add State(s) to Queue__JKI_lib_State_Machine.vi"("State(s) in Front (\"\")"="//Exit Sub-Modules ", "State(s) in (\"\")"=w349, "State(s) at Back (\"\")"="Data: Cleanup\nExit") -> ("States Out"=w351:string)  [unwired: 12 in]
                n106 = call <vilib>:"Add State(s) to Queue__JKI_lib_State_Machine.vi"("State(s) in Front (\"\")"=w351, "State(s) in (\"\")"=w356) -> ("States Out"=w355:string)  [unwired: 13 in]
              }
              frame "---------- API ----------" {
                # "#CSM \"Category Seperator\"\nDo not put any code in this frame."
              }
              frame "API: API1" {
                # "#CSM API Example\nCopy/Rename this case for your own API"
                # "#CSM Response\nConnect this to return the response of your API"
                # "#CSM >> Msg/Rep's CSM >>\nIf you need to tell who triggered this state , use this string. If it's this case itself, this string is \"\"."
                # "#CSM >> Arguments >>\nDeal with the parameter if any"
              }
              frame "API: API2" {
                # "#CSM API Example\nCopy/Rename this case for your own API"
                # "unpack Hex String  to Variant\nif complex parameter is needed."
                n107 = call "CSM - Convert HexStr to Data.vi"("HEX String"=w365) -> ()  [unwired: 7 in, 2 out]
                n108 = disable-structure shown="Disabled" {
                  disable-tunnel: [w369 "API2 Response"] -> w364
                  frame Disabled {
                    # "pack variant to hexstr \nif complex response is needed."
                    # "complex Response"
                    n109 = call "CSM - Convert Data to HexStr.vi"() -> ("HEX String (0-9,A-F)"=w369:string)  [unwired: 9 in]
                  }
                  frame Enabled {
                  }
                }
              }
              frame "---------- Action ----------" {
                # "#CSM \"Category Seperator\"\nDo not put any code in this frame."
                n110 = call <vilib>:"Add State(s) to Queue__JKI_lib_State_Machine.vi"("State(s) in (\"\")"=w374) -> ("States Out"=w373:string)  [unwired: 14 in]
              }
              frame "Action: action1" {
                # "#CSM \"Internal State\"\nThis category is used for holding internal states"
                n111 = call <vilib>:"Add State(s) to Queue__JKI_lib_State_Machine.vi"("State(s) in (\"\")"=w378) -> ("States Out"=w377:string)  [unwired: 14 in]
              }
              frame "Action: action2" {
                # "#CSM \"Internal State\"\nThis category is used for holding internal states"
                n112 = call <vilib>:"Add State(s) to Queue__JKI_lib_State_Machine.vi"("State(s) in (\"\")"=w382) -> ("States Out"=w381:string)  [unwired: 14 in]
              }
            }
          }
          n113 = for {
            shift-right: [w85] -> w61
            shift-left: w60 -> [w86]
            shift-right: [w87] -> w66
            shift-left: w67 -> [w88]
            tunnel: w65 -> [w99] mode=indexing
            i -> [w101]
            stop <- w84 stop-if-true
            w79 = "Handler Message" ("To")
            n114 = Unbundle By Name(w99) -> ("From"=w97:string, "To"=w93:string)
            n115 = Increment(x=w101) -> (x+1=→"LoopCount 2":i32)
            n116 = call "uuid.vi"() -> ("UUID"=w90:string)  [unwired: 11 in]
            n117 = call "CSM - Wait and Send Message for Reply.vi"("State"="API: Test Register Status", "Arguments (\"\")"=w90, "Target Module"=w97) -> ("error out"=w96:errorcluster)  [unwired: 9 in, 3 out]
            n118 = call "Stall Data Flow.vim"("value in"=w96, "milliseconds to wait"=u32 100) -> ("value out"=w94:errorcluster)  [unwired: 1 out]
            n119 = call "CSM Get Module Attribute.vim"("CSM Name"=w93, "Attribute"=w79, "Default Value (Empty Variant)"="", "Error In"=w94) -> ("CSM Name (Dup)"=w80:string, "Found"=w92:bool, "Value"=w89:string, "error out"=w81:errorcluster)  [unwired: 7 in, 1 out]
            n120 = Equal?(x=w90, y=w89) -> (x = y?=w83:bool)
            n121 = flat-sequence {
              tunnel: w81 -> [w104]
              tunnel: w80 -> [w103]
              tunnel: w79 -> [w102]
              frame #0 {
                n122 = call <vilib>:"Clear Errors.vi"("error in (no error)"=w104) -> ("error out"=w105:errorcluster)  [unwired: 5 in, 1 out]
                n123 = call "CSM - Delete Module Attribute.vi"("CSM Name"=w103, "Attribute"=w102, "Error In"=w105) -> ()  [unwired: 9 in, 4 out]
              }
            }
            n124 = And(x=w92, y=w83) -> (x .and. y?=w82:bool)
            n125 = call-dynamic "passIf.vi"("error in (no error)"=w86, "pass"=w82, "TestCase in"=w88) -> ("error out"=w85:errorcluster, "TestCase out"=w87:refnum<class "testcase-CSMBroadcast.lvclass">)  [unwired: 7 in]
            n126 = Unbundle By Name(w85) -> ("status"=w84:bool)
          }
          n127 = flat-sequence {
            tunnel: w62 -> [w73]
            tunnel: w61 -> [w72]
            tunnel: [w71] -> w56
            tunnel: w56 -> [w78]
            tunnel: [w77] -> w55
            frame #0 {
              n128 = call "CSM - Send Message and Wait for Reply.vi"("Target Module"=w73, "State"="Macro: Exit") -> ("error out"=w75:errorcluster)  [unwired: 7 in, 2 out]
              n129 = Merge Errors(w72, w75) -> (w71:errorcluster)
            }
            frame #1 {
              n130 = call "CSM - Drop Broadcast Registry.vi"() -> ("error out"=w76:errorcluster)  [unwired: 15 in]
              n131 = Merge Errors(w78, w76) -> (w77:errorcluster)
            }
          }
        }
      }
    }
    frame Disabled {
      # "skip test result while test is under development"
      n132 = call <vilib>:"skip.vi"("error in (no error)"=w383, "TestCase in"=w386) -> ("error out"=w385:errorcluster, "TestCase out"=w384:refnum<class "testcase-CSMBroadcast.lvclass">)  [unwired: 8 in]
    }
  }
  "error out" <- w3
  "TestCase out" <- w1
